vi "Test2(ByValue)_Init.vi"(0 "object in":refnum<class "Test2(ByValue).lvclass">, 2 "TestName":string, 5 "error in (no error)":errorcluster) -> (14 "object out":refnum<class "Test2(ByValue).lvclass">, 19 "error out":errorcluster)   [LabVIEW 2016, in "Test2(ByValue).lvclass"]
uses:
  Test2(ByValue).lvclass
  Test2(ByValue).lvclass/Test2(ByValue).ctl
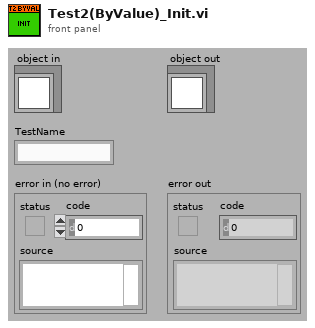
[diagram p1: front panel]
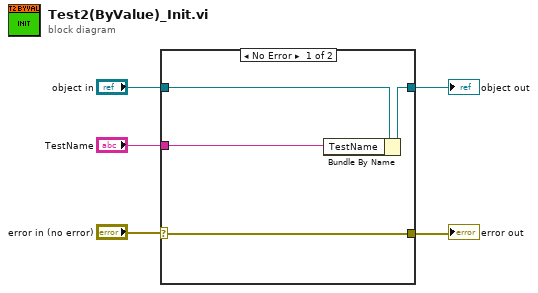
[diagram p0: block diagram]
diagram:
  n1 = case shown="No Error" "error in (no error)" {
    selector: "error in (no error)" -> [w7 w10]
    tunnel: "object in" -> [w9 w11]
    tunnel: [w8 w11] -> w4
    tunnel: [w7 w10] -> w2
    tunnel: "TestName" -> [w6 _]
    frame No Error {
      n2 = Bundle By Name(cluster=w9, "TestName"=w6) -> (w8:refnum<class "Test2(ByValue).lvclass">)
    }
    frame Error {
    }
  }
  "object out" <- w4
  "error out" <- w2
